vi "Run_Calibration_Matlab.vi"(3 "Show Matlab":bool, 4 "Cal Level":dbl, 5 "Selection String":string) -> (0 "EVM Pre-Cal":dbl, 2 "EVM Post-Cal":dbl)   [LabVIEW 2024]
panel:
  out "standard output":string
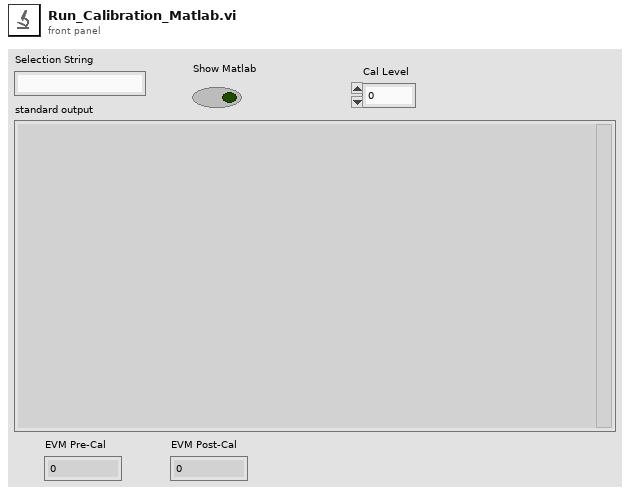
[diagram p1: front panel]
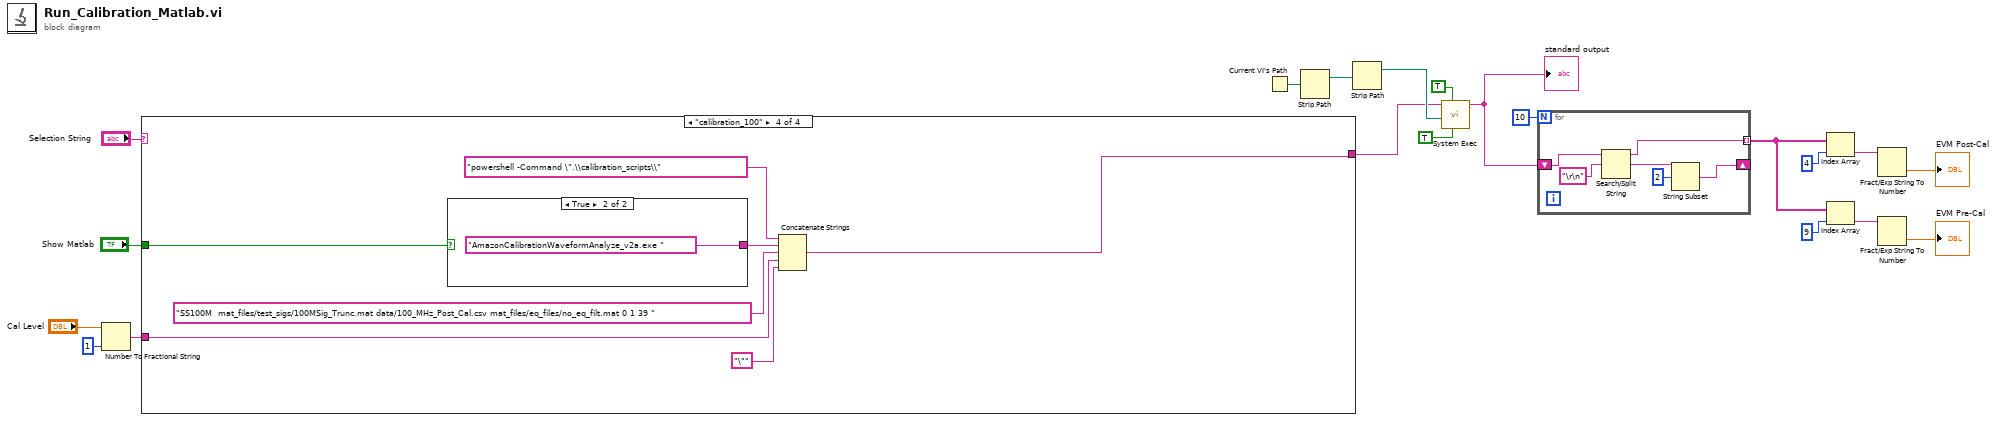
[diagram p0: block diagram]
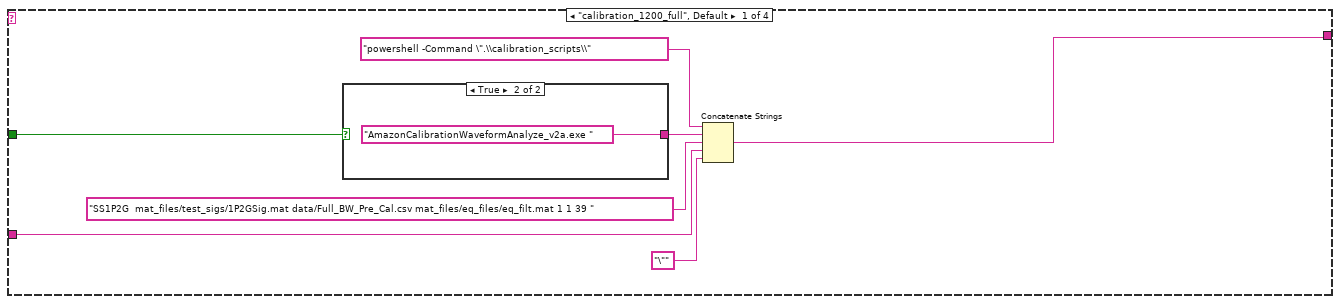
[diagram p2: hidden frame]
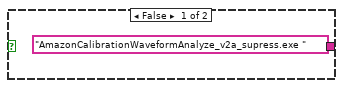
[diagram p3: hidden frame]
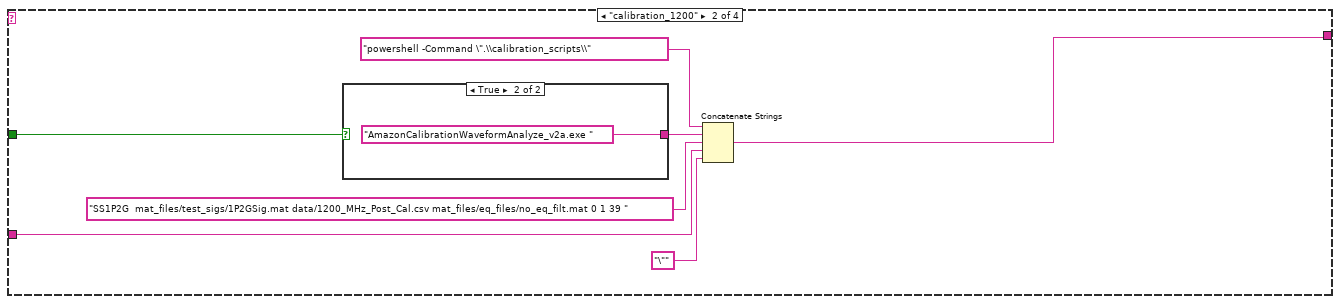
[diagram p4: hidden frame]
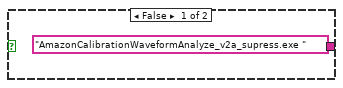
[diagram p5: hidden frame]
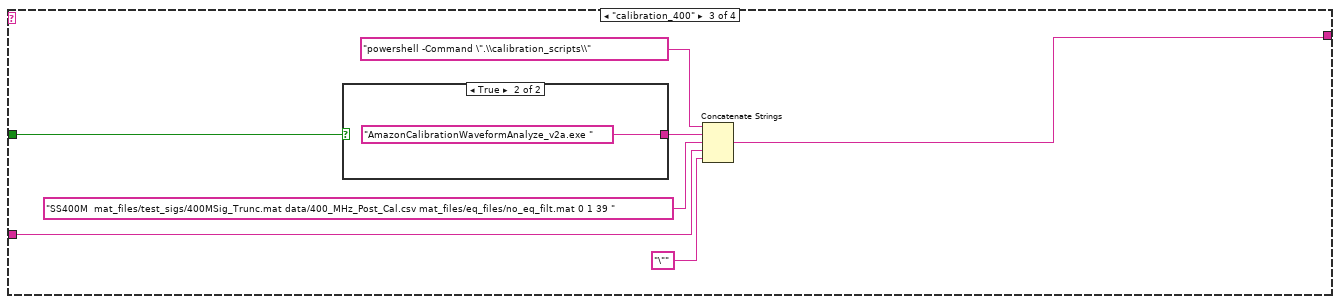
[diagram p6: hidden frame]
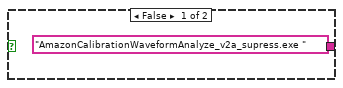
[diagram p7: hidden frame]
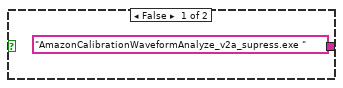
[diagram p8: hidden frame]
diagram:
  n1 = Number To Fractional String(number="Cal Level", precision (6)=i16 1) -> (F-format string=w2:string)  [unwired: 2 in]
  n2 = case shown="\"calibration_100\"" "Selection String" {
    tunnel: [w24 w33 w42 w51] -> w6
    tunnel: w2 -> [w22 w31 w40 w49]
    tunnel: "Show Matlab" -> [w21 w30 w39 w48]
    frame "calibration_1200_full", Default {
      n3 = case shown="True" w21 {
        tunnel: ["AmazonCalibrationWaveformAnalyze_v2a_supress.exe " "AmazonCalibrationWaveformAnalyze_v2a.exe "] -> w26
        frame False {
        }
        frame True {
        }
      }
      n4 = Concatenate Strings("powershell -Command \".\\calibration_scripts\\" ("command line"), w26, "SS1P2G  mat_files/test_sigs/1P2GSig.mat data/Full_BW_Pre_Cal.csv mat_files/eq_files/eq_filt.mat 1 1 39 " ("command line"), w22, "\"" ("command line")) -> (w24:string)
    }
    frame "calibration_1200" {
      n5 = case shown="True" w30 {
        tunnel: ["AmazonCalibrationWaveformAnalyze_v2a_supress.exe " "AmazonCalibrationWaveformAnalyze_v2a.exe "] -> w35
        frame False {
        }
        frame True {
        }
      }
      n6 = Concatenate Strings("powershell -Command \".\\calibration_scripts\\" ("command line"), w35, "SS1P2G  mat_files/test_sigs/1P2GSig.mat data/1200_MHz_Post_Cal.csv mat_files/eq_files/no_eq_filt.mat 0 1 39 " ("command line"), w31, "\"" ("command line")) -> (w33:string)
    }
    frame "calibration_400" {
      n7 = case shown="True" w39 {
        tunnel: ["AmazonCalibrationWaveformAnalyze_v2a_supress.exe " "AmazonCalibrationWaveformAnalyze_v2a.exe "] -> w44
        frame False {
        }
        frame True {
        }
      }
      n8 = Concatenate Strings("powershell -Command \".\\calibration_scripts\\" ("command line"), w44, "SS400M  mat_files/test_sigs/400MSig_Trunc.mat data/400_MHz_Post_Cal.csv mat_files/eq_files/no_eq_filt.mat 0 1 39 " ("command line"), w40, "\"" ("command line")) -> (w42:string)
    }
    frame "calibration_100" {
      n9 = case shown="True" w48 {
        tunnel: ["AmazonCalibrationWaveformAnalyze_v2a_supress.exe " "AmazonCalibrationWaveformAnalyze_v2a.exe "] -> w53
        frame False {
        }
        frame True {
        }
      }
      n10 = Concatenate Strings("powershell -Command \".\\calibration_scripts\\" ("command line"), w53, "SS100M  mat_files/test_sigs/100MSig_Trunc.mat data/100_MHz_Post_Cal.csv mat_files/eq_files/no_eq_filt.mat 0 1 39 " ("command line"), w49, "\"" ("command line")) -> (w51:string)
    }
  }
  n11 = Current VI's Path() -> (path=w19:path)
  n12 = Strip Path(path=w19) -> (stripped path=w18:path)  [unwired: 1 out]
  n13 = Strip Path(path=w18) -> (stripped path=w17:path)  [unwired: 1 out]
  n14 = call <vilib>:"System Exec.vi"("run minimized? (F)"=TRUE, "wait until completion? (T)"=TRUE, "working directory"=w17, "command line"=w6) -> ("standard output"=w11:string)  [unwired: 4 in, 3 out]
  "standard output" <- w11
  n15 = for {
    N: 10 -> [_]
    shift-right: [w57] -> _
    shift-left: w11 -> [w61]
    tunnel: [w60] -> w7 mode=indexing
    n16 = Search/Split String(string=w61, search string/char (-)="\r\n") -> (substring before match=w60:string, match + rest of string=w59:string)  [unwired: 1 in, 1 out]
    n17 = String Subset(string=w59, offset (0)=2) -> (substring=w57:string)  [unwired: 1 in]
  }
  n18 = Index Array(array=w7, index=4) -> (element=w13:string)
  n19 = Index Array(array=w7, index=9) -> (element=w9:string)
  n20 = Fract/Exp String To Number(string=w13) -> (number=→"EVM Post-Cal":dbl)  [unwired: 3 in, 1 out]
  n21 = Fract/Exp String To Number(string=w9) -> (number=→"EVM Pre-Cal":dbl)  [unwired: 3 in, 1 out]
